vi "Write connection.vi"(8 "error in (no error)":errorcluster, 10 "connection":refnum<k24>, 11 "DbConnection in":refnum<class "ORM_DBC_dotNet.lvclass">) -> (0 "error out":errorcluster, 3 "DbConnection out":refnum<class "ORM_DBC_dotNet.lvclass">)   [LabVIEW 2020, in "ORM_DBC_dotNet.lvlib" / "ORM_DBC_dotNet.lvclass"]
uses:
  ORM_DBC_dotNet.lvclass
  System.Data
  ORM_DBC_dotNet.lvclass/ORM_DBC_dotNet.ctl
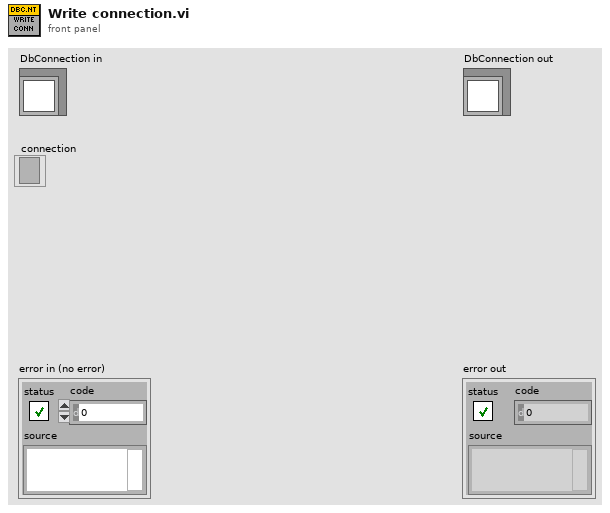
[diagram p1: front panel]
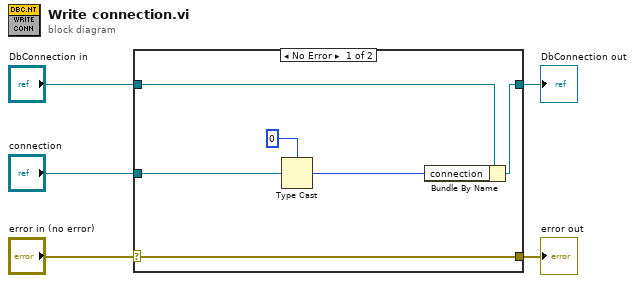
[diagram p0: block diagram]
diagram:
  n1 = case shown="No Error" "error in (no error)" {
    selector: "error in (no error)" -> [w11 w12]
    tunnel: [w11 w12] -> w4
    tunnel: [w9 w13] -> w2
    tunnel: "DbConnection in" -> [w10 w13]
    tunnel: "connection" -> [w8 _]
    frame No Error {
      n2 = Type Cast(type=u64 0 ("connection"), x=w8) -> (*(type *) &x=w6:u64)
      n3 = Bundle By Name(cluster=w10, "connection"=w6) -> (w9:refnum<class "ORM_DBC_dotNet.lvclass">)
    }
    frame Error {
    }
  }
  "error out" <- w4
  "DbConnection out" <- w2
